vi "Post Substeps PWM Output Task.vi"(8 "error in":errorcluster, 9 "PWM Output In":T1, 10 "Socket No":u16=1, 11 "Sequence Context In":refnum<k7>) -> (0 "error out":errorcluster, 3 "Report Text":string)   [LabVIEW 2023, in "LTT_TeststandSteptypes.lvlib"]
doc: "This VI Is Socket Number based AO Data Signal Write Through Q"
uses:
  LTT_TeststandSteptypes.lvlib
  HardwareAbstractionLayer_LVOOP/PWM Output/NI PWM Output_class/NI PWM DAQ/Control/PWM Output Edit.ctl
  HardwareAbstractionLayer_LVOOP/PWM Output/NI PWM Output_class/NI PWM Output.lvclass
  HardwareAbstractionLayer_LVOOP/Teststand/Teststand Engine Driver/Control/Teststand Status Control.ctl
  HardwareAbstractionLayer_LVOOP/Main/Main.lvclass
  HardwareAbstractionLayer_LVOOP/Main/Class Options.ctl
  <vilib>/Utility/error.llb/DialogType.ctl
  <resource>/objmgr/daqmx.rc
  <vilib>/DAQmx/create/channels.llb/DAQmx Create Channel (CO-Pulse Generation-Frequency).vi
  <vilib>/DAQmx/configure/timing.llb/DAQmx Timing (Implicit).vi
  HardwareAbstractionLayer_LVOOP/Database/Database.lvclass
  HardwareAbstractionLayer_LVOOP/Database/SQL Public VI/Control/DB Options.ctl
  HardwareAbstractionLayer_LVOOP/PWM Output/PWM Output_class/PWM Output.lvclass
  HardwareAbstractionLayer_LVOOP/Teststand/Teststand.lvclass
panel:
  in  "stop":bool
  out "error out 2":errorcluster
  out "Actual Frequency":dbl[](array[numeric])
  out "Actual Duty Cycle":dbl[](array[numeric])
  in  "Stop":bool
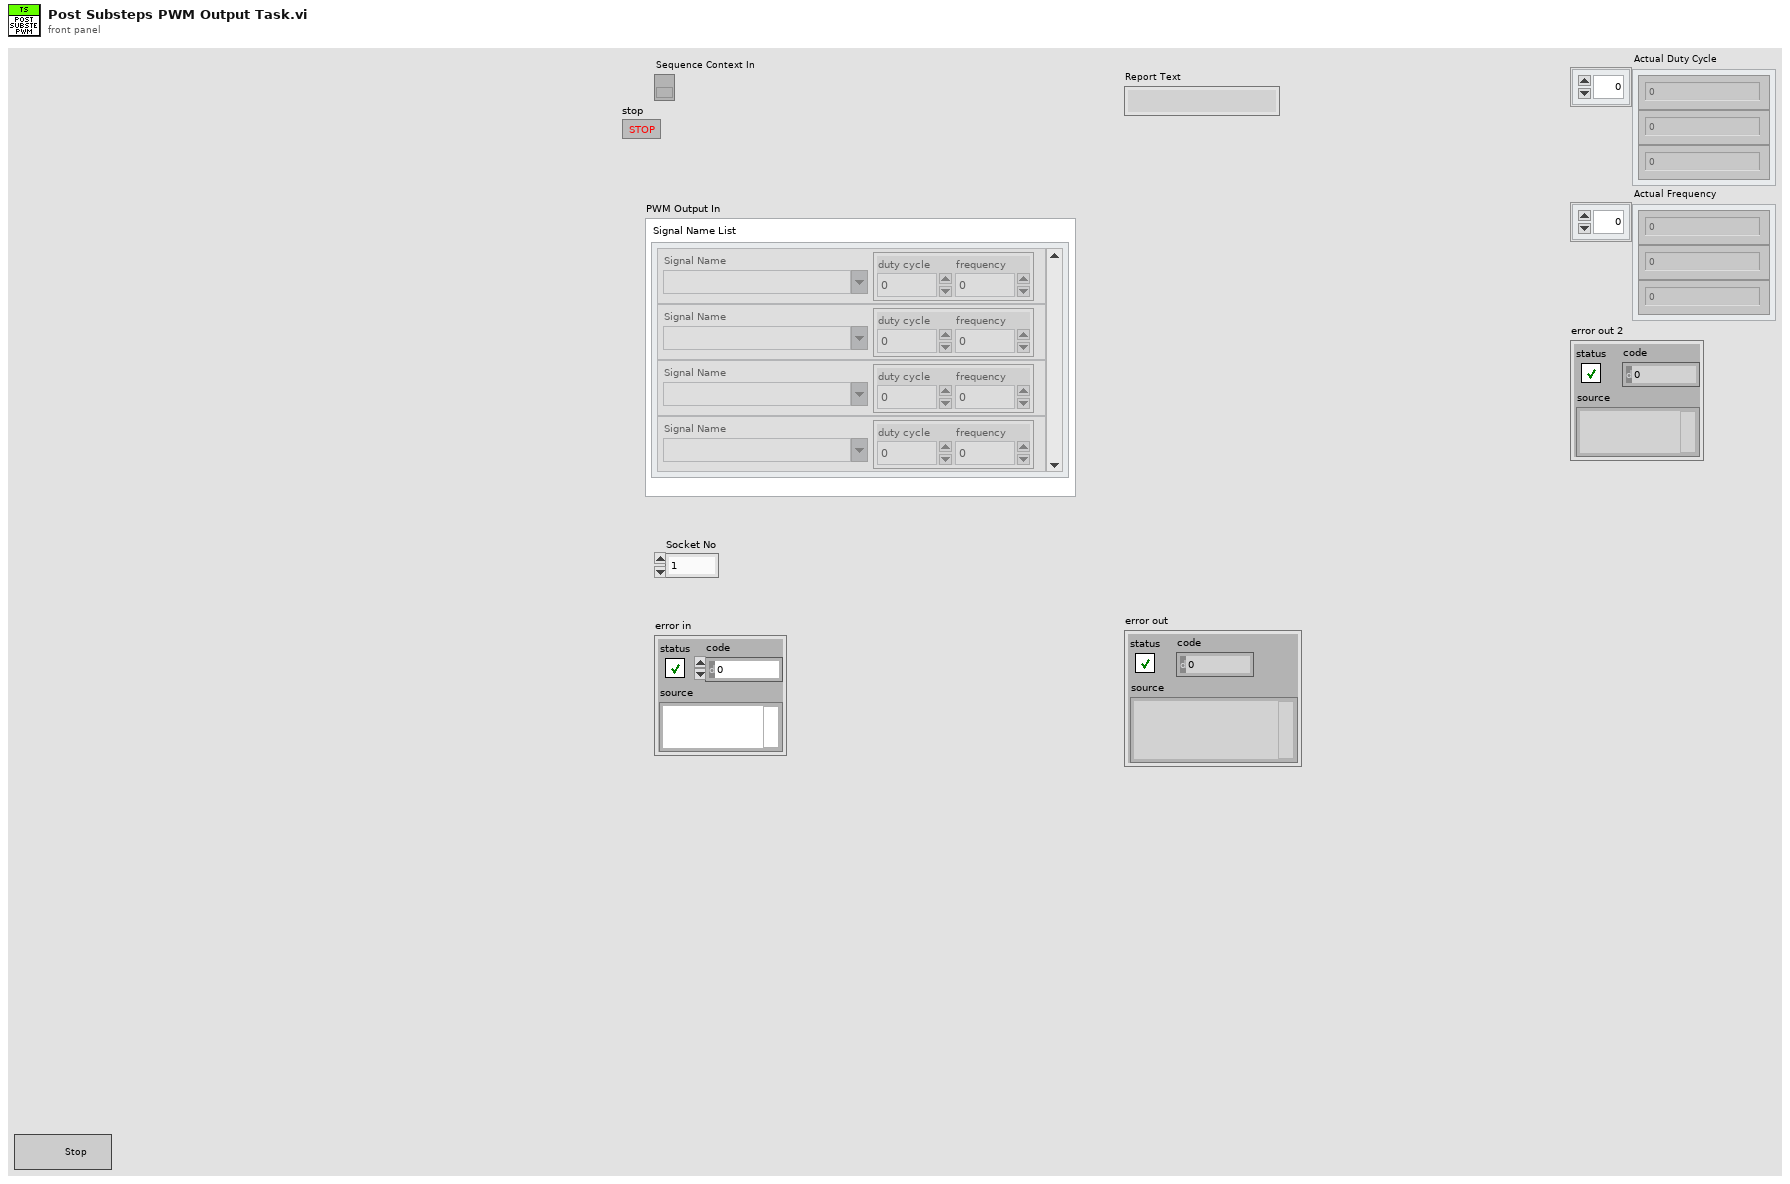
[diagram p1: front panel]
types:
  T1 = typedef "HardwareAbstractionLayer_LVOOP.lvlib/NI PWM Output.lvclass/PWM Output Edit.ctl" = cluster{"Signal Name List":cluster{"Signal Name":string, "values":cluster{"duty cycle":dbl, "frequency":dbl}}[]}
  T2 = typedef "HardwareAbstractionLayer_LVOOP.lvlib/Teststand.lvclass/Teststand Status Control.ctl" = cluster{"Terminating or Aborting":bool, "Stop":bool, "Socket Count":i16, "Selected Sockets":i16[]}
  T3 = typedef "HardwareAbstractionLayer_LVOOP.lvlib/Main.lvclass/Class Options.ctl" = enum16{"Init All Class", "Read All Class", "Write AI Class", "Write AO Class", "Write AO Waveform Generation", "Write DI Class", "Write DO Class", "Write PWM Input Class", "Write PWM Output Class", "Exit"}
  T4 = typedef "HardwareAbstractionLayer_LVOOP.lvlib/Main.lvclass/Class Ref.ctl" = cluster{"FGV":refnum<class "Function Global Variable.lvclass">, "Notifier":refnum<class "NotifierHandler.lvclass">, "Queue":refnum<class "Queue Handler.lvclass">, "User Event":refnum<class "User Event.lvclass">, "Data Manager":refnum<class "Data Manager.lvclass">, "DMM":refnum<class "DMM.lvclass">, "Function Generator":refnum<class "Function Generator.lvclass">, "Oscilloscope":refnum<class "Oscilloscope.lvclass">, "PowerSupply":refnum<class "PowerSupply.lvclass">, "Teststand":refnum<class "Teststand.lvclass">, "AO":refnum<class "AO.lvclass">, "AI":refnum<class "AI.lvclass">, "Database":refnum<class "Database.lvclass">, "AO Waveform Generation":refnum<class "AO.lvclass">, "DO":refnum<class "DO.lvclass">, "DI":refnum<class "DI.lvclass">, "PWM Output":refnum<class "PWM Output.lvclass">, "PWM Input":refnum<class "PWM Input.lvclass">, "RelayOutput":refnum<class "NISwitch.lvclass">, "Modbus":refnum<class "Modbus.lvclass">, "CAN":refnum<class "CAN.lvclass">}
  T5 = typedef "DialogType.ctl" = u16
  T6 = typedef "HardwareAbstractionLayer_LVOOP.lvlib/Database.lvclass/DB Options.ctl" = enum16{"Init", "Select Data", "Insert Data", "Update Data", "Delete Data", "Execute Query", "Create Schema", "Create Table", "List Tables", "List Columns", "Close"}
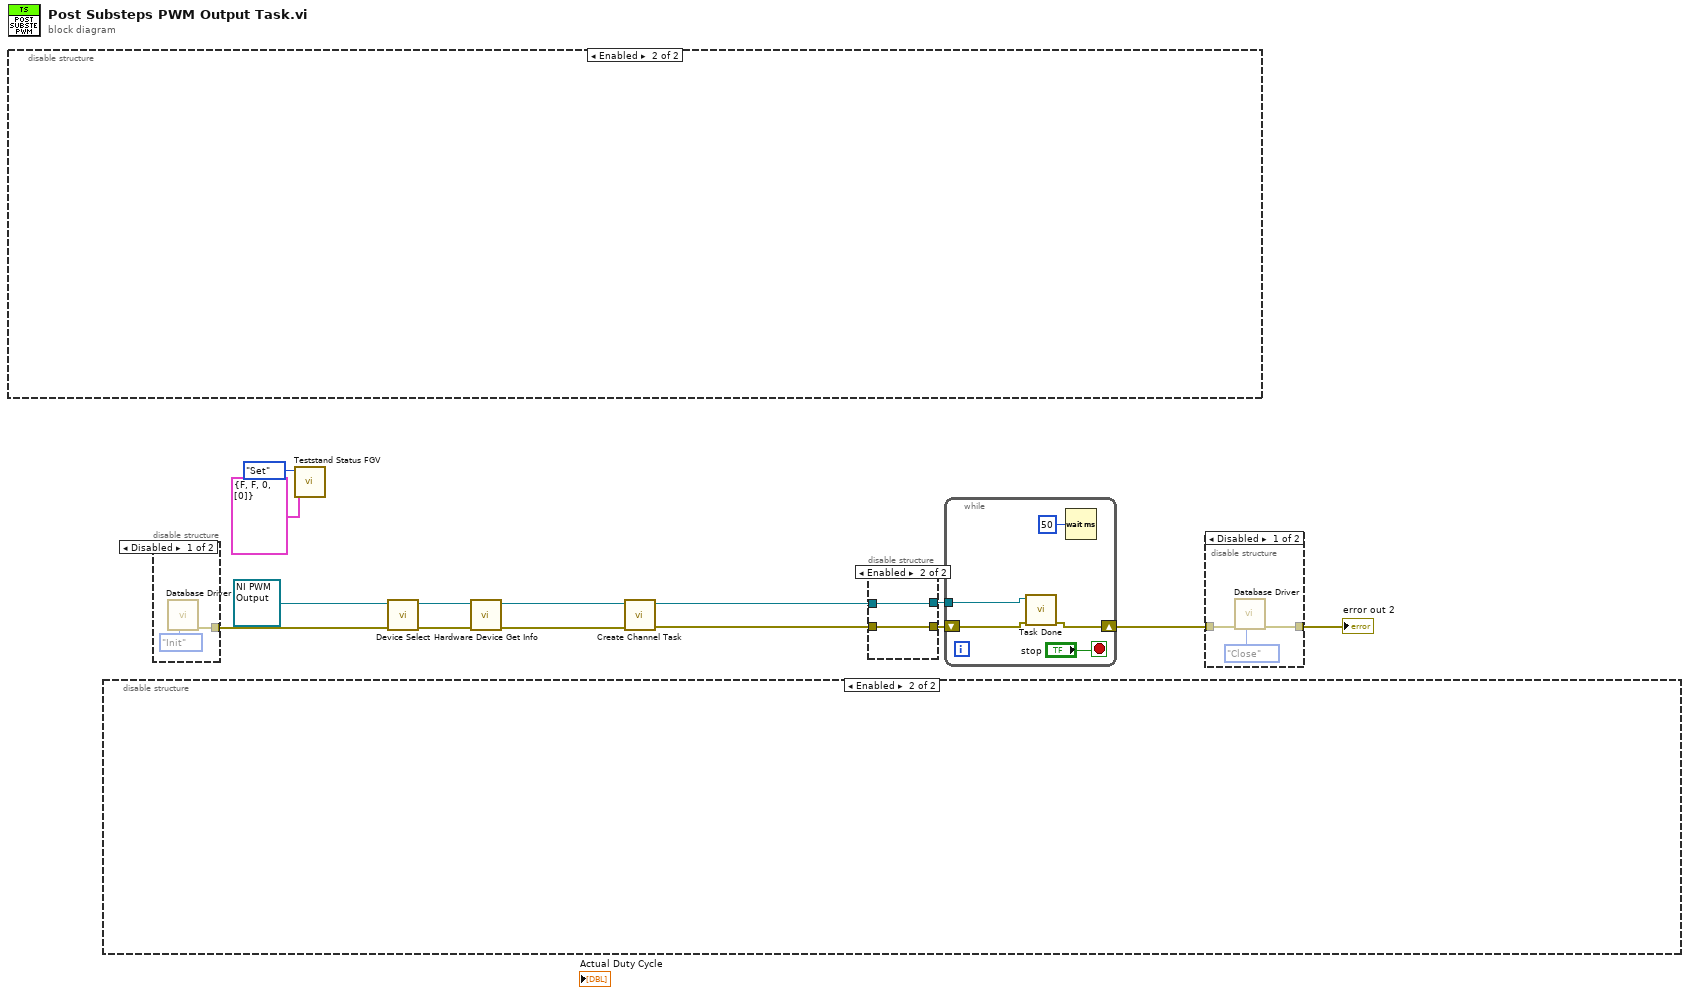
[diagram p0: block diagram]
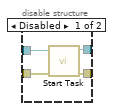
[diagram p4: hidden frame]
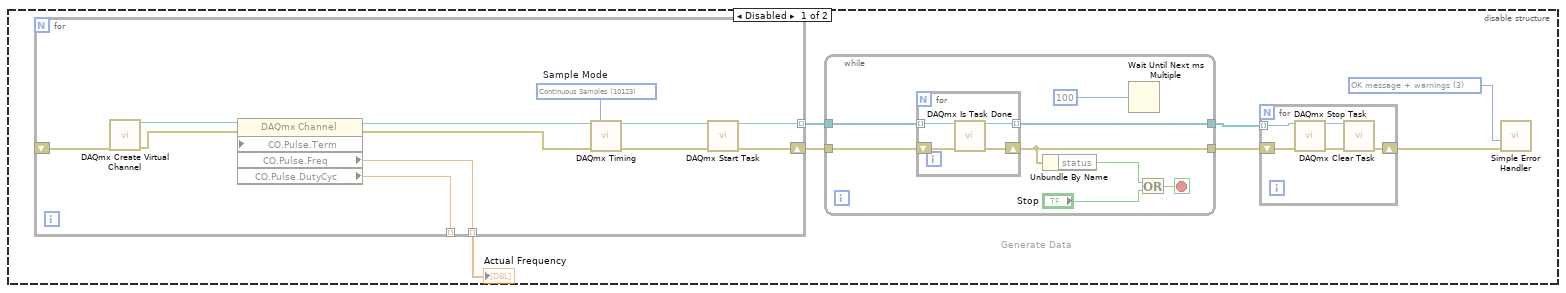
[diagram p5: hidden frame]
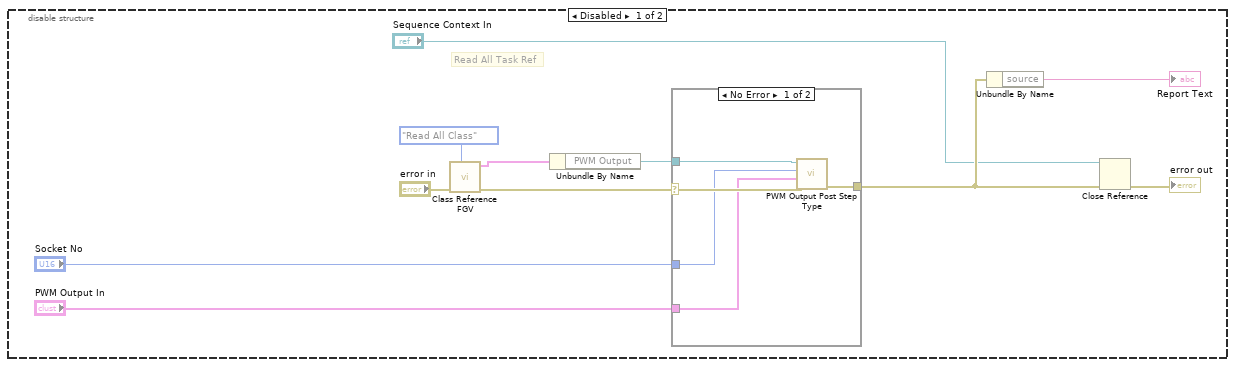
[diagram p6: hidden frame]
diagram:
  n1 = disable-structure shown="Enabled" {
    frame Disabled {
      # "Read All Task Ref"
      n2 = call "Class Reference FGV.vi"("Options"=Class_Options."Read All Class", "error in"="error in") -> ("error out"=w19:errorcluster, "Class Cluster Out"=w17:T4)  [unwired: 8 in]
      n3 = Unbundle By Name(w17) -> ("PWM Output"=w16:refnum<class "PWM Output.lvclass">)
      n4 = case shown="No Error" w19 {
        selector: w19 -> [w29 w31]
        tunnel: [w28 w31] -> w25
        tunnel: "PWM Output In" -> [w26 _]
        tunnel: "Socket No" -> [w27 _]
        tunnel: w16 -> [w30 _]
        frame No Error {
          n5 = call-dynamic "PWM Output Post Step Type.vi"("error in (no error)"=w29, "PWM Output In"=w26, "Socket No"=w27, "PWM Output in"=w30) -> ("error out"=w28:errorcluster)  [unwired: 6 in, 1 out]
        }
        frame Error {
        }
      }
      n6 = Unbundle By Name(w25) -> ("source"=→"Report Text":string)
      n7 = Close Reference(reference="Sequence Context In", error in (no error)=w25) -> (error out=→"error out":errorcluster)
    }
    frame Enabled {
    }
  }
  n8 = disable-structure shown="Enabled" {
    frame Disabled {
      w34 = T5 3 items=["no dialog", "OK message", "continue or stop message", "OK message + warnings", "continue/stop + warnings"] ("type of dialog (OK msg:1)")
      # "Generate Data"
      n9 = for {
        tunnel: [w54] -> w38 mode=indexing
        tunnel: [w46] -> w33 mode=indexing
        tunnel: [w45] -> _ mode=indexing
        shift-right: [w53] -> w37
        shift-left: _ -> [w44]
        w55 = 10123 items=["Finite Samples"=10178, "Continuous Samples"=10123, "Hardware Timed Single Point"=12522]  # Sample Mode
        n10 = call-poly <vilib>:"DAQmx Create Virtual Channel.vi"("error in"=w44) -> ("task out"=w50:refnum<k21>, "error out"=w49:errorcluster)  [unwired: 13 in]
        n11 = property class="DAQmx Channel" props=["CO.Pulse.Term", "CO.Pulse.Freq", "CO.Pulse.DutyCyc"](reference=w50, error in=w49) -> (reference out=w47:refnum<k21>, error out=w48:errorcluster, "CO.Pulse.Freq"=w46:dbl, "CO.Pulse.DutyCyc"=w45:dbl)  [unwired: 1 in]
        n12 = call-poly <vilib>:"DAQmx Timing.vi"("task/channels in"=w47, "sample mode"=w55, "error in"=w48) -> ("task out"=w51:refnum<k21>, "error out"=w52:errorcluster)  [unwired: 11 in]
        n13 = call <vilib>:"DAQmx Start Task.vi"("task/channels in"=w51, "error in"=w52) -> ("task out"=w54:refnum<k21>, "error out"=w53:errorcluster)  [unwired: 12 in]
      }
      "Actual Frequency" <- w33
      n14 = while {
        tunnel: w38 -> [w56]
        tunnel: w37 -> [w63]
        tunnel: [w60] -> w35
        tunnel: [w61] -> w32
        stop <- w62 stop-if-true
        n15 = for {
          tunnel: [w66] -> w61 mode=indexing
          shift-right: [w65] -> w60
          shift-left: w63 -> [w67]
          tunnel: w56 -> [w64] mode=indexing
          n16 = call <vilib>:"DAQmx Is Task Done.vi"("task/channels in"=w64, "error in"=w67) -> ("task out"=w66:refnum<k21>, "error out"=w65:errorcluster)  [unwired: 11 in, 1 out]
        }
        n17 = Unbundle By Name(w60) -> ("status"=w59:bool)
        n18 = Wait Until Next ms Multiple(millisecond multiple=u32 100) -> ()  [unwired: 1 out]
        n19 = Or(x=w59, y="Stop") -> (x .or. y?=w62:bool)
      }
      n20 = for {
        shift-right: [w43] -> w36
        shift-left: w35 -> [w40]
        tunnel: w32 -> [w39] mode=indexing
        n21 = call <vilib>:"DAQmx Stop Task.vi"("task/channels in"=w39, "error in"=w40) -> ("task out"=w42:refnum<k21>, "error out"=w41:errorcluster)  [unwired: 12 in]
        n22 = call <vilib>:"DAQmx Clear Task.vi"("task in"=w42, "error in"=w41) -> ("error out"=w43:errorcluster)  [unwired: 13 in]
      }
      n23 = call <vilib>:"Simple Error Handler.vi"("type of dialog (OK msg:1)"=w34, "error in (no error)"=w36) -> ()  [unwired: 3 in, 5 out]
    }
    frame Enabled {
    }
  }
  n24 = disable-structure shown="Disabled" {
    disable-tunnel: [w68 _] -> w7
    frame Disabled {
      n25 = call "Database Driver.vi"("Options"=DB_Options."Init") -> ("error out"=w68:errorcluster)  [unwired: 7 in, 3 out]
    }
    frame Enabled {
    }
  }
  n26 = call "Teststand Status FGV.vi"("Teststand Status"=T2 {"Terminating or Aborting"=FALSE, "Stop"=FALSE, "Socket Count"=0, "Selected Sockets"=[0]}, "Option"=enum16{"Set", "Get"}."Set") -> ()  [unwired: 8 in, 2 out]
  n27 = call-dynamic "Device Select.vi"("error in"=w7, "NI PWM Output in"=refnum<class "NI PWM Output.lvclass"> refnum ("HardwareAbstractionLayer_LVOOP.lvlib:NI PWM Output.lvclass")) -> ("error out"=w12:errorcluster, "NI PWM Output out"=w13:refnum<class "NI PWM Output.lvclass">)  [unwired: 8 in]
  n28 = call-dynamic "Hardware Device Get Info.vi"("error in"=w12, "NI PWM Output in"=w13) -> ("error out"=w10:errorcluster, "NI PWM Output out"=w11:refnum<class "NI PWM Output.lvclass">)  [unwired: 8 in]
  n29 = call-dynamic "Create Channel Task.vi"("error in"=w10, "NI PWM Output in"=w11) -> ("error out"=w8:errorcluster, "NI PWM Output out"=w9:refnum<class "NI PWM Output.lvclass">)  [unwired: 8 in]
  n30 = disable-structure shown="Enabled" {
    disable-tunnel: w9 -> [w73 w75]
    disable-tunnel: w8 -> [w72 w74]
    disable-tunnel: [w71 w75] -> w5
    disable-tunnel: [w70 w74] -> w4
    frame Disabled {
      n31 = call-dynamic "Start Task.vi"("error in"=w72, "NI PWM Output in"=w73) -> ("error out"=w70:errorcluster, "NI PWM Output out"=w71:refnum<class "NI PWM Output.lvclass">)  [unwired: 8 in]
    }
    frame Enabled {
    }
  }
  n32 = while {
    tunnel: w5 -> [w80]
    shift-right: [w78] -> w3
    shift-left: w4 -> [w79]
    stop <- "stop" stop-if-true
    n33 = call-dynamic "Task Done.vi"("error in (no error)"=w79, "NI PWM Output in"=w80) -> ("error out"=w78:errorcluster)  [unwired: 8 in, 1 out]
    n34 = Wait (ms)(milliseconds to wait=u32 50) -> ()  [unwired: 1 out]
  }
  n35 = disable-structure shown="Disabled" {
    disable-tunnel: [w83 _] -> w6
    disable-tunnel: w3 -> [w81 _]
    frame Disabled {
      n36 = call "Database Driver.vi"("Options"=DB_Options."Close", "error in"=w81) -> ("error out"=w83:errorcluster)  [unwired: 6 in, 3 out]
    }
    frame Enabled {
    }
  }
  "error out 2" <- w6
